vi "VI_PowerSpectrum.v1.1.vi"() -> ()   [LabVIEW 2018]
uses:
  <vilib>/Analysis/2dsp.llb/Real FFT.vi
  <vilib>/measure/maspectr.llb/FFT Power Spectrum and PSD for 1 Chan.vi
  <vilib>/rtlsdr/rtlsdr.lvlib
  <vilib>/measure/NI_MAPro.lvlib
  <vilib>/Analysis/NI_AALPro.lvlib
panel:
  out "FFT":cluster{dbl[], "FFT {X}":dbl[]}(graph)
  out "Power Spectrum":cluster{"f0":dbl, "df":dbl, "magnitude":dbl[]}(graph)
  out "Center Frequency":dbl
  in  "config":bool
  in  "Number Of Samples":i32
  in  "Center Frequency":u32
  in  "Sample Rate":u32
  out "function return":i32
  in  "Device Index":u32
  out "Device USB Strings":T1
  out "DeviceRefnum Out":u64
  in  "stop":bool
  out "Device Count":u32
  # "1"
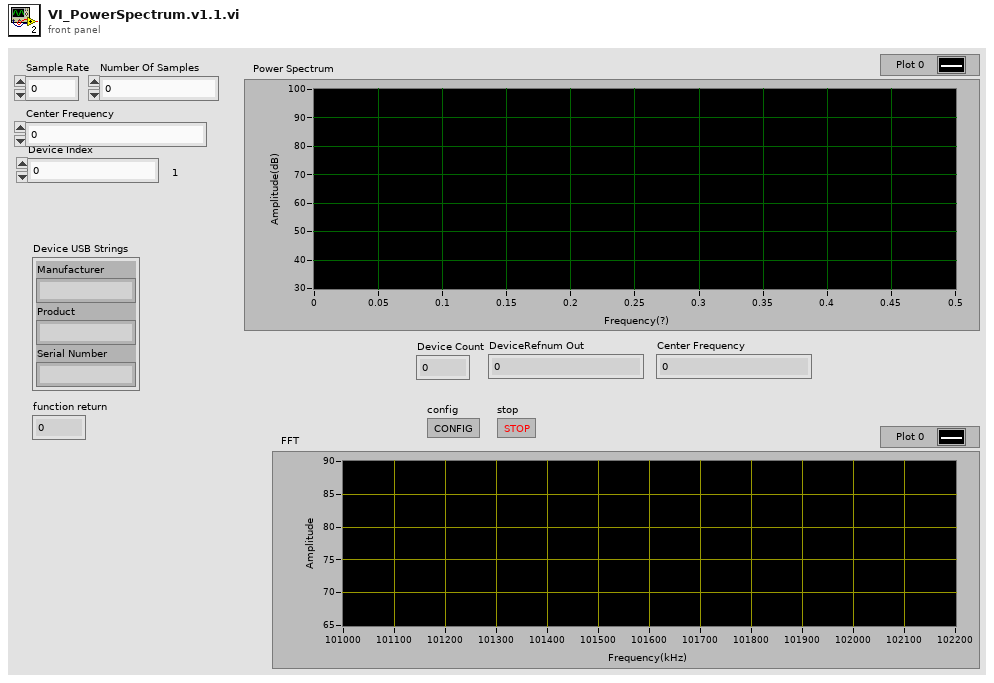
[diagram p1: front panel]
types:
  T1 = cluster{"Manufacturer":string, "Product":string, "Serial Number":string}
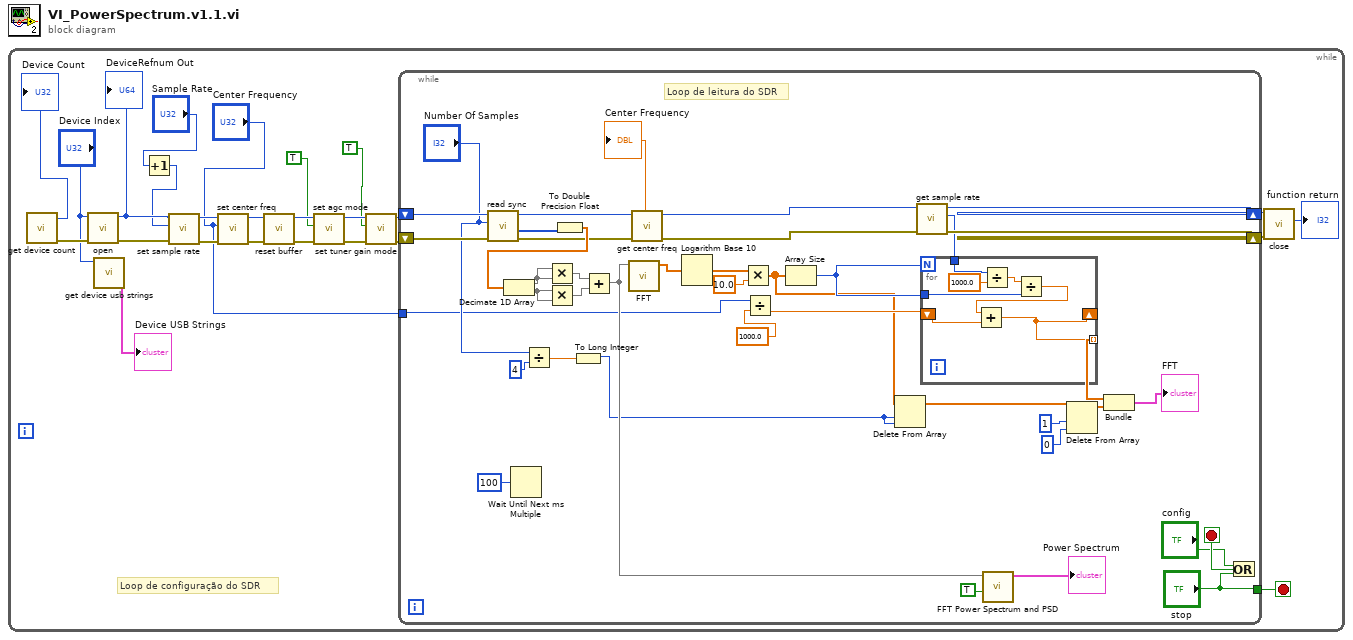
[diagram p0: block diagram]
diagram:
  n1 = while {
    stop <- w5 stop-if-true
    # "Loop de configuração do SDR"
    n2 = call <vilib>:"get device count.vi"() -> ("error out"=w24:errorcluster, "Device Count"=→"Device Count":u32)  [unwired: 10 in]
    n3 = call <vilib>:"open.vi"("error in (no error)"=w24, "Device Index"="Device Index") -> ("error out"=w20:errorcluster, "DeviceRefnum Out"=w19:u64)  [unwired: 6 in]
    "DeviceRefnum Out" <- w19
    n4 = call <vilib>:"get device usb strings.vi"("Device Index"="Device Index") -> ("Device USB Strings"=→"Device USB Strings":T1)  [unwired: 8 in, 2 out]
    n5 = Increment(x="Sample Rate") -> (x+1=w3:u32)
    n6 = call <vilib>:"set sample rate.vi"("error in (no error)"=w20, "Sample Rate"=w3, "DeviceRefnum"=w19) -> ("error out"=w18:errorcluster, "DeviceRefnum Out"=w17:u64)  [unwired: 6 in, 1 out]
    n7 = call <vilib>:"set center freq.vi"("error in (no error)"=w18, "Center Frequency"="Center Frequency", "DeviceRefnum"=w17) -> ("error out"=w16:errorcluster, "DeviceRefnum Out"=w15:u64)  [unwired: 6 in, 1 out]
    n8 = call <vilib>:"reset buffer.vi"("error in (no error)"=w16, "DeviceRefnum"=w15) -> ("error out"=w14:errorcluster, "DeviceRefnum Out"=w13:u64)  [unwired: 7 in, 1 out]
    n9 = call <vilib>:"set agc mode.vi"("error in (no error)"=w14, "AGC Enable"=TRUE, "DeviceRefnum"=w13) -> ("error out"=w12:errorcluster, "DeviceRefnum Out"=w11:u64)  [unwired: 6 in, 1 out]
    n10 = call <vilib>:"set tuner gain mode.vi"("error in (no error)"=w12, "AutoGain"=TRUE ("AGC Enable"), "DeviceRefnum"=w11) -> ("error out"=w9:errorcluster, "DeviceRefnum Out"=w8:u64)  [unwired: 6 in, 1 out]
    n11 = while {
      shift-right: [w36] -> w6
      shift-left: w8 -> [w65]
      shift-right: [w37] -> w7
      shift-left: w9 -> [w66]
      tunnel: ["stop"] -> w5
      tunnel: "Center Frequency" -> [w41]
      stop <- w61 stop-if-true
      # "Loop de leitura do SDR"
      n12 = call <vilib>:"read sync.vi"("error in (no error)"=w66, "Number Of Samples"="Number Of Samples", "DeviceRefnum"=w65) -> ("error out"=w39:errorcluster, "Sample Buffer"=w63:u8[], "DeviceRefnum Out"=w58:u64)  [unwired: 5 in, 1 out]
      n13 = Wait Until Next ms Multiple(millisecond multiple=u32 100) -> ()  [unwired: 1 out]
      n14 = Divide(x="Number Of Samples", y=4) -> (x/y=w48:dbl)
      n15 = To Double Precision Float(number=w63) -> (double precision float=w64:dbl[])
      n16 = Decimate 1D Array(w64) -> (w56:dbl[], w55:dbl[])
      n17 = Multiply(x=w56, y=w56) -> (x*y=w54:dbl[])
      n18 = Multiply(x=w55, y=w55) -> (x*y=w53:dbl[])
      n19 = To Long Integer(number=w48) -> (32bit integer=w34:i32)
      n20 = Add(x=w54, y=w53) -> (x+y=w50:dbl[])
      n21 = call-poly <vilib>:"FFT.vi"("X"=w50) -> ("FFT {X}"=w29:cdb[])  [unwired: 9 in, 1 out]
      n22 = call <vilib>:"get center freq.vi"("error in (no error)"=w39, "DeviceRefnum"=w58) -> ("error out"=w38:errorcluster, "Center Frequency"=→"Center Frequency":dbl, "DeviceRefnum Out"=w40:u64)  [unwired: 7 in]
      n23 = Logarithm Base 10(1:w29) -> (0:w27:cdb[])
      n24 = Multiply(x=w27, y=10.0) -> (x*y=w28:cdb[])
      n25 = Divide(x=w41, y=1000.0) -> (x/y=w43:dbl)
      n26 = Array Size(array=w28) -> (size(s)=w47:i32)
      n27 = Delete From Array(array=w28, length=w34, index=w34) -> (array with subset deleted=w33:cdb[])  [unwired: 1 out]
      n28 = call <vilib>:"get sample rate.vi"("error in (no error)"=w38, "DeviceRefnum"=w40) -> ("error out"=w37:errorcluster, "Sample Rate (Hz)"=w35:u32, "DeviceRefnum Out"=w36:u64)  [unwired: 7 in]
      n29 = for {
        N: w47 -> [_]
        tunnel: w47 -> [w73]
        shift-right: [w70] -> _
        shift-left: w43 -> [w72]
        tunnel: [w70] -> w46 mode=indexing
        tunnel: w35 -> [w67]
        n30 = Divide(x=w67, y=1000.0) -> (x/y=w69:dbl)
        n31 = Divide(x=w69, y=w73) -> (x/y=w71:dbl)
        n32 = Add(x=w71, y=w72) -> (x+y=w70:dbl)
      }
      n33 = call-poly <vilib>:"FFT Power Spectrum and PSD.vi"("dB On (F)"=TRUE, "time signal"=w50) -> ("Power Spectrum / PSD"=→"Power Spectrum":cluster{"f0":dbl, "df":dbl, "magnitude":dbl[]})  [unwired: 6 in, 3 out]
      n34 = Delete From Array(array=w33, length=1, index=0) -> (array with subset deleted=w32:cdb[])  [unwired: 1 out]
      n35 = Bundle(w46, w32) -> (→"FFT":cluster{dbl[], cdb[]})  [unwired: 1 in]
      n36 = Or(x="config", y="stop") -> (x .or. y?=w61:bool)
    }
    n37 = call <vilib>:"close.vi"("error in (no error)"=w7, "DeviceRefnum"=w6) -> ("function return"=→"function return":i32)  [unwired: 8 in, 1 out]
  }
